vi "readMotorPodMisc.vi"(8 "error in (no error)":errorcluster, 9 "Input Pod Clustor":T1, 10 "Pod Number":i32, 11 "Refnum in":T2) -> (1 "output cluster":T1)   [LabVIEW 2014]
uses:
  <vilib>/Utility/config.llb/Config Data RefNum.ctl
  read/readDoubleKey.vi
  read/readI32.vi
  <vilib>/Utility/config.llb/NI_LVConfig.lvlib
panel:
  out "Refnum out":T2
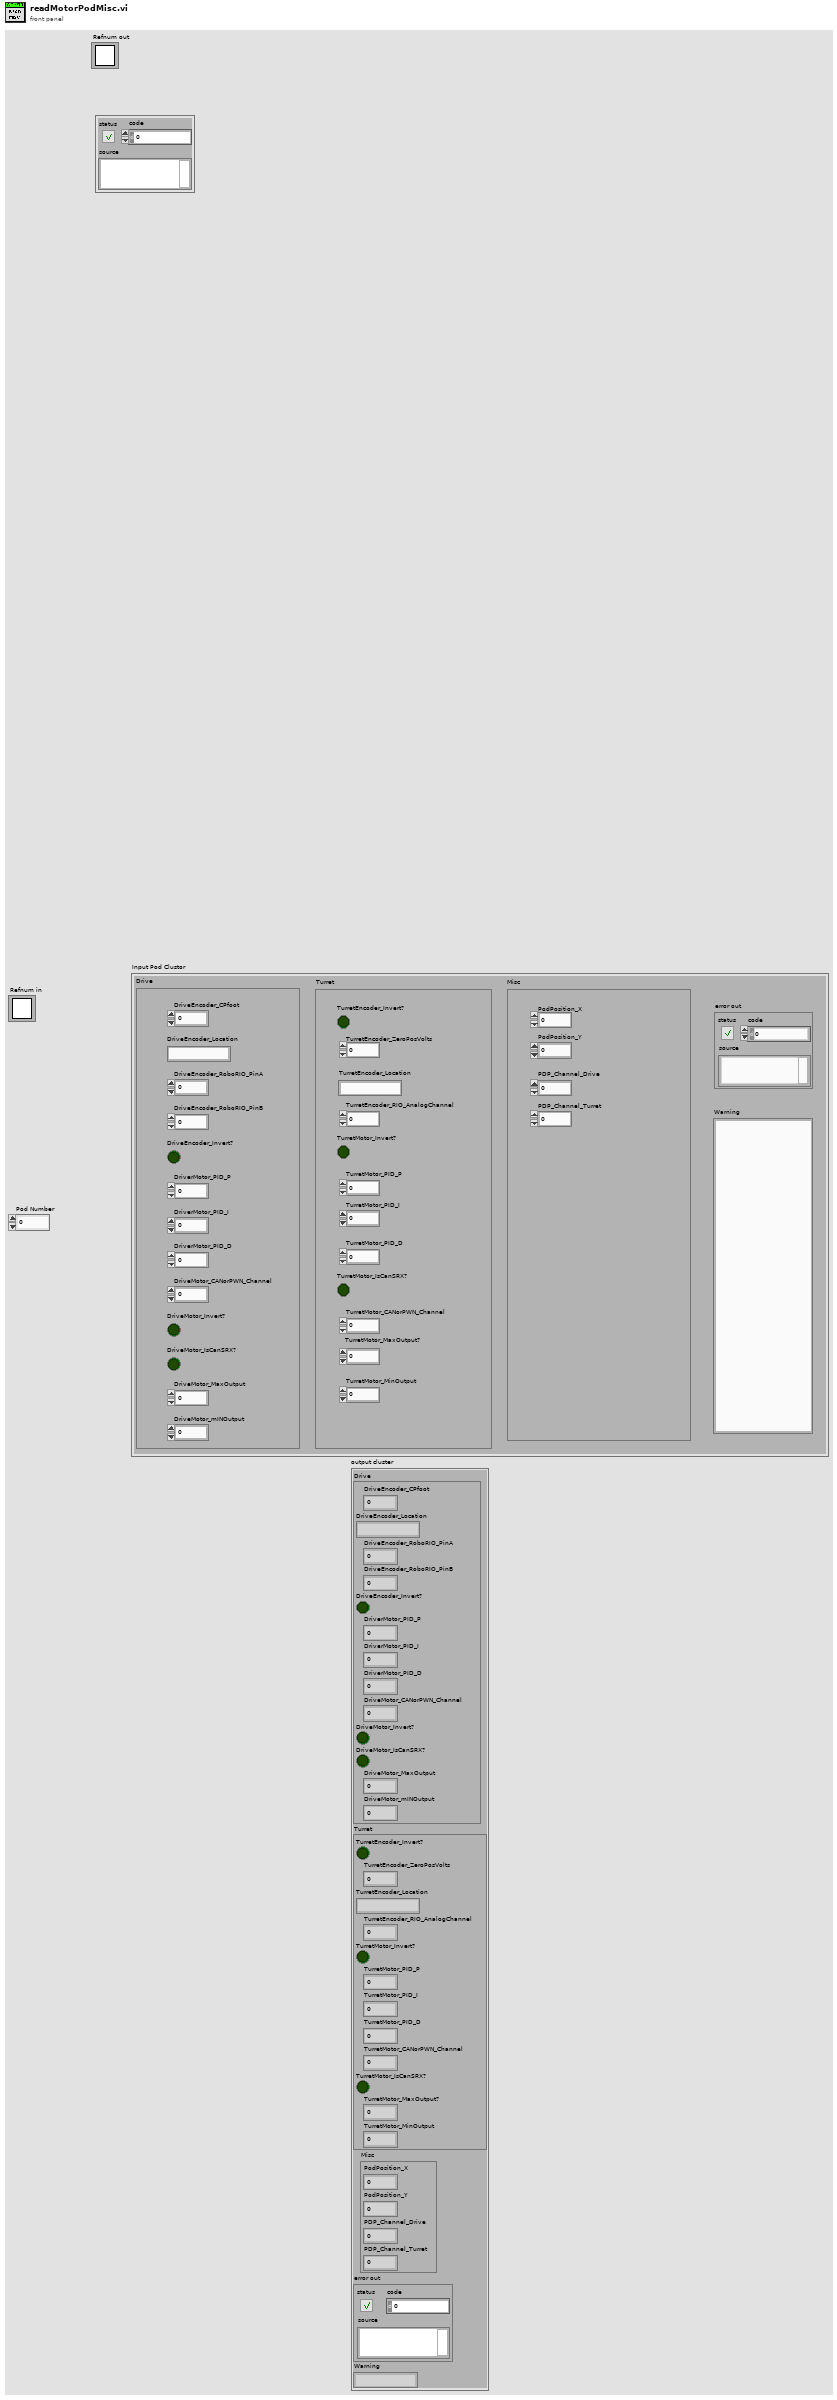
[diagram p1: front panel]
types:
  T1 = cluster{"Drive":cluster{"DriveEncoder_CPfoot":dbl, "DriveEncoder_Location":string, "DriveEncoder_RoboRIO_PinA":i32, "DriveEncoder_RoboRIO_PinB":i32, "DriveEncoder_Invert?":bool, "DriverMotor_PID_P":dbl, "DriverMotor_PID_I":dbl, "DriverMotor_PID_D":dbl, "DriveMotor_CANorPWN_Channel":i32, "DriveMotor_Invert?":bool, "DriveMotor_IsCanSRX?":bool, "DriveMotor_MaxOutput":dbl, "DriveMotor_mINOutput":dbl}, "Turret":cluster{"TurretEncoder_Invert?":bool, "TurretEncoder_ZeroPosVolts":dbl, "TurretEncoder_Location":string, "TurretEncoder_RIO_AnalogChannel":dbl, "TurretMotor_Invert?":bool, "TurretMotor_PID_P":dbl, "TurretMotor_PID_I":dbl, "TurretMotor_PID_D":dbl, "TurretMotor_CANorPWN_Channel":dbl, "TurretMotor_IsCanSRX?":bool, "TurretMotor_MaxOutput?":dbl, "TurretMotor_MinOutput":dbl}, "Misc":cluster{"PodPosition_X":dbl, "PodPosition_Y":dbl, "PDP_Channel_Drive":i32, "PDP_Channel_Turret":i32}, "error out":errorcluster, "Warning":string}
  T2 = typedef "NI_LVConfig.lvlib/Config Data RefNum.ctl" = refnum<k1>
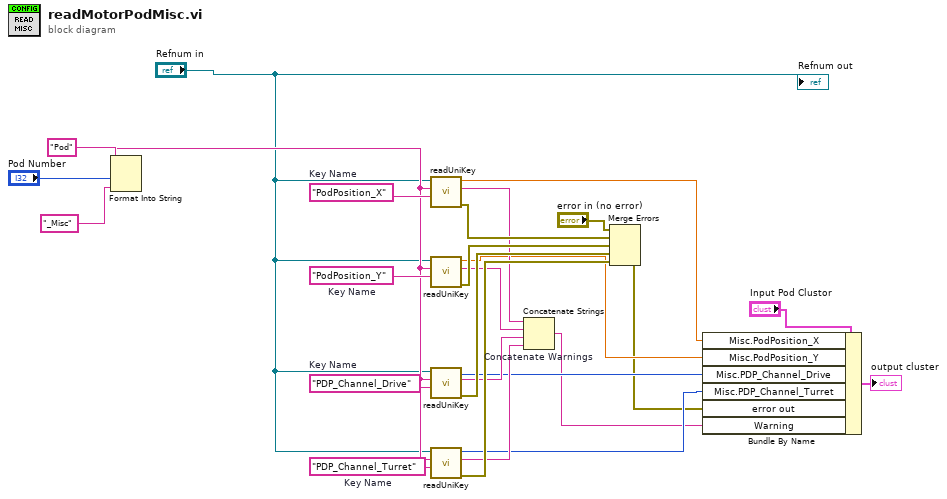
[diagram p0: block diagram]
diagram:
  w24 = "PDP_Channel_Turret"  # Key Name
  w23 = "PDP_Channel_Drive"  # Key Name
  w25 = "PodPosition_Y"  # Key Name
  w26 = "PodPosition_X"  # Key Name
  n1 = Format Into String(initial string="Pod", "Pod Number", "_Misc") -> (resulting string=w13:string)  [unwired: 2 in, 1 out]
  n2 = call-poly "readUniKey.vi"("Refnum in"="Refnum in", "Section"=w13, "Key Name"=w26) -> ("value"=w7:dbl, "Warning"=w18:string, "error out"=w22:errorcluster)  [unwired: 5 in]
  n3 = call-poly "readUniKey.vi"("Refnum in"="Refnum in", "Section"=w13, "Key Name"=w25) -> ("value"=w6:dbl, "Warning"=w17:string, "error out"=w21:errorcluster)  [unwired: 5 in]
  n4 = call-poly "readUniKey.vi"("Refnum in"="Refnum in", "Section"=w13, "Key Name"=w23) -> ("value"=w5:i32, "Warning"=w16:string, "error out"=w20:errorcluster)  [unwired: 5 in]
  n5 = call-poly "readUniKey.vi"("Refnum in"="Refnum in", "Section"=w13, "Key Name"=w24) -> ("value"=w4:i32, "Warning"=w15:string, "error out"=w19:errorcluster)  [unwired: 5 in]
  n6 = Concatenate Strings "Concatenate Warnings"(w18, w17, w16, w15) -> (w2:string)
  n7 = Merge Errors "Merge Errors"("error in (no error)", w22, w21, w20, w19) -> (w3:errorcluster)
  n8 = Bundle By Name(cluster="Input Pod Clustor", "Misc.PodPosition_X"=w7, "Misc.PodPosition_Y"=w6, "Misc.PDP_Channel_Drive"=w5, "Misc.PDP_Channel_Turret"=w4, "error out"=w3, "Warning"=w2) -> (→"output cluster":T1)
  "Refnum out" <- "Refnum in"
